vi "StopData.vi"(8 "error in (no error)":errorcluster, 11 "Class In":refnum<class "C37.118 Sim.lvclass">) -> (0 "error out":errorcluster, 3 "Class Out":refnum<class "C37.118 Sim.lvclass">)   [LabVIEW 2014, in "SensorPlugins.lvlib" / "C37.118 Sim.lvclass"]
uses:
  C37.118 Sim.lvclass
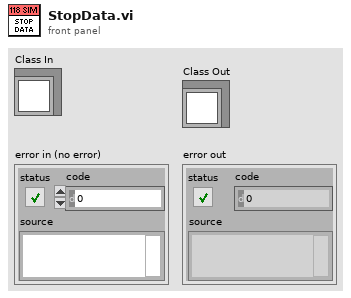
[diagram p1: front panel]
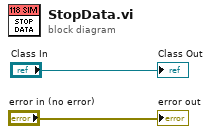
[diagram p0: block diagram]
diagram:
  "Class Out" <- "Class In"
  "error out" <- "error in (no error)"
